vi "Close Device Editor UI.vi"(5 "Save":bool, 7 "Notifier":refnum<notifier>, 10 "error in (no error)":errorcluster, 11 "Close Event":refnum<user-event>) -> (2 "error out":errorcluster, 3 "Aborted":bool)   [LabVIEW 2012, in "HAL Config.lvlib" / "HAL Editor.lvclass"]
uses:
  HAL Editor.lvclass
  build/ppl/lv-hal.lvlibp/Device/Editor Event Data.ctl
  build/ppl/lv-hal.lvlibp/Device/Device.lvclass
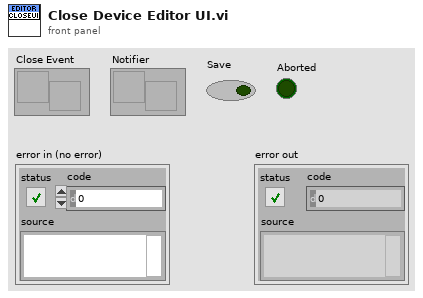
[diagram p1: front panel]
types:
  T1 = typedef "lv-hal.lvlibp/Device.lvclass/Editor Event Data.ctl" = cluster{"Save":bool, "Done Notifier":refnum<notifier>}
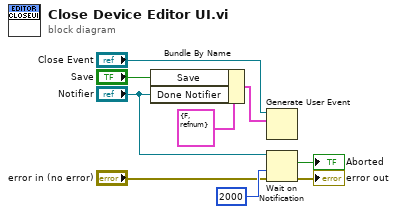
[diagram p0: block diagram]
diagram:
  n1 = Bundle By Name(cluster=T1 {"Save"=FALSE, "Done Notifier"=refnum} ("event data"), "Save"="Save", "Done Notifier"="Notifier") -> (w8:T1)
  n2 = Generate User Event(user event="Close Event", event data cluster=w8) -> ()  [unwired: 1 in, 2 out]
  n3 = Wait on Notification(notifier="Notifier", timeout in ms (-1)=2000, error in (no error)="error in (no error)") -> (notification=→"Aborted":bool, error out=→"error out":errorcluster)  [unwired: 1 in, 2 out]
